vi "NI 9411_TASK_COUNT.vi"(6 "divisor":u32=4, 8 "error in":errorcluster, 9 "CI.Freq.Term":tag="/CDRMod7/PFI3", 11 "MODULE NAME":string="cDAQ_NICOTRAMod5/ctr0") -> (0 "error out":errorcluster, 3 "task out":refnum<k21>)   [LabVIEW 2016]
uses:
  <vilib>/DAQmx/create/channels.llb/DAQmx Create Channel (CI-Frequency).vi
  <resource>/objmgr/daqmx.rc
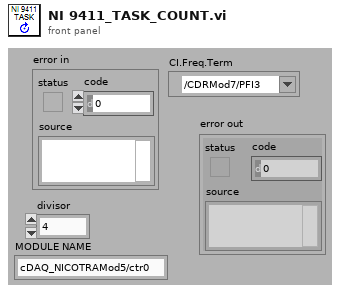
[diagram p1: front panel]
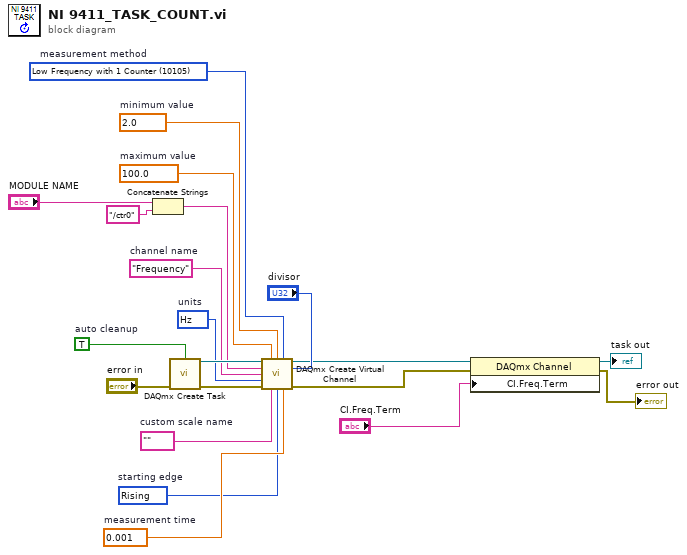
[diagram p0: block diagram]
diagram:
  w4 = tag ""  # custom scale name
  w5 = 10280 items=["Rising"=10280, "Falling"=10171]  # starting edge
  w11 = 10373 items=["Hz"=10373, "Ticks"=10304, "From Custom Scale"=10065]  # units
  w12 = 0.001  # measurement time
  w14 = 10105 items=["Low Frequency with 1 Counter"=10105, "High Frequency with 2 Counters"=10157, "Large Range with 2 Counters"=10205]  # measurement method
  w15 = "Frequency"  # channel name
  w16 = 2.0  # minimum value
  w17 = 100.0  # maximum value
  w19 = TRUE  # auto cleanup
  n1 = Concatenate Strings("MODULE NAME", "/ctr0" ("string")) -> (w8:string)
  n2 = call <vilib>:"DAQmx Create Task.vi"("auto cleanup"=w19, "error in"="error in") -> ("task out"=w18:refnum<k21>, "error out"=w20:errorcluster)  [unwired: 12 in]
  n3 = call-poly <vilib>:"DAQmx Create Virtual Channel.vi"("task in"=w18, "maximum value"=w17, "minimum value"=w16, "measurement method"=w14, "counter"=w8, "divisor"="divisor", "name to assign"=w15, "units"=w11, "error in"=w20, "custom scale name"=w4, "starting edge"=w5, "measurement time"=w12) -> ("task out"=w7:refnum<k21>, "error out"=w3:errorcluster)  [unwired: 2 in]
  n4 = property class="DAQmx Channel"(reference=w7, error in=w3, "CI.Freq.Term"="CI.Freq.Term") -> (reference out=→"task out":refnum<k21>, error out=→"error out":errorcluster)
